vi "Recursive Model&Adaptive Control.vi"() -> ()   [LabVIEW 2015]
uses:
  <vilib>/addons/Control Design/_Model Construction/Model Typedefs.llb/CD State Space Model (MIMO).ctl
  <vilib>/addons/Control Design/_Model Construction/Model Typedefs.llb/CD General Elements.ctl
  <vilib>/addons/Control Design/_Stochastic Systems/Stochastic Systems.llb/Stochastic Systems SubVIs/cd_Second-Order Statistics Noise Model.ctl
  <vilib>/Platform/TimedLoop/XDataNode/timing_clust.ctl
  <vilib>/Platform/TimedLoop/XDataNode/nitl_modes.ctl
  <vilib>/Platform/TimedLoop/XDataNode/wakeup.ctl
  <vilib>/addons/Control Design/_Model Construction/Model Creation.llb/Model Creation SubVI/cd_Create State Space Model.vi
  <vilib>/FPGAPlugInAG/myRIO-1900/niLvFpga_Open_myRIO-1900.vi
  <vilib>/rvi/interface/common/dynamic/niFpgaDynamicAddResources.vi
  <vilib>/Utility/error.llb/Error Cluster From Error Code.vi
  <vilib>/rvi/errors/niLvFpgaAdjustHostInterfaceError.vi
  <vilib>/FPGAPlugInAG/Dynamic/niLvFpga_Close_Dynamic.vi
  <vilib>/addons/Control Design/_State Feedback Control/State Feedback Control.llb/State Feedback Control SubVis/cd_Kalman Gain (Stochastic).vi
  <vilib>/addons/Control Design/_State Feedback Control/State Feedback Control.llb/State Feedback Control SubVis/cd_Linear Quadratic Regulator.vi
  <vilib>/addons/Control Design/_State Feedback Control/State Feedback Control.llb/CD State Regulator.vi
  <vilib>/addons/Control Design/_Model Construction/Model Information.llb/Model Information SubVIs/cd_Get Matrices From SS Model.vi
  <vilib>/rvi/interface/nirviOpenFPGA/nirviOpenFPGA.xnode
  FPGA Bitfiles/ACC20115_FPGATarget_CurrentControlle_Dt5vFgOzYtY.lvbitx
  Current Controller.vi
  <vilib>/rvi/interface/nirviReadWriteControl/nirviReadWriteControl.xnode
  <vilib>/rvi/interface/nirviCloseFPGA/nirviCloseFPGA.xnode
  <vilib>/Platform/TimedLoop/XDataNode/XDataNode.xnode
  NiFpgaLv.dll
  <vilib>/rvi/interface/Simulation/niFpgaSimulationCallBeginRW.vi
  <vilib>/addons/Control Design/_Stochastic Systems/NI_CD_Stochastic Systems.lvlib
  <vilib>/Platform/TimedLoop/XDataNode/XDNodeRunTimeDep.lvlib
  <vilib>/addons/Control Design/_Model Construction/NI_LinSys_Model Creation.lvlib
  <vilib>/addons/Control Design/_State-Space Analysis/NI_CD_State-Space Analysis.lvlib
  <vilib>/addons/Control Design/_State Feedback Control/NI_CD_State Feedback Control.lvlib
  <vilib>/addons/Control Design/_Model Construction/NI_LinSys_Model Information.lvlib
  <vilib>/addons/Control Design/_Model Construction/NI_LinSys_Model Typedefs.lvlib
panel:
  out "error IO":errorcluster
  in  "Tab Control":enum32{"Outputs/Control", "Model Info"}(tab)
  out "DAC Inlet Valve 2":i32(graph)
  out "Fusion Data":dbl(graph)
  in  "Stop":bool
  out "FPGA Status?":bool
  in  "Current (mA)":i32
  out "Priori SS Detectable?":bool
  out "Priori SS Observable?":bool
  out "State-Space Model":T1 {"Transport Delay" format="%.2f"; "D" format="%#.2g"; "C" format="%#.2g"; "B" format="%#.2g"; "A" format="%#.2g"; "properties"."Sampling Time" format="%#.6p"; "properties"."Output Delays" format="%.4f"; "properties"."Input Delays" format="%.4f"}
  in  "A":dbl[][](array[numeric]) format="%#.5g"
  in  "B":dbl[][](array[numeric]) format="%#.5g"
  in  "C":dbl[][](array[numeric]) format="%#.5g"
  in  "D":dbl[][](array[numeric]) format="%#.5g"
  in  "G":dbl[][](array[numeric]) format="%#.2g"
  out "Riccati Solution (X)":dbl[][](array[numeric]) format="%.4f"
  in  "Noise Model":T3 {"N" format="%#.2g"; "R" format="%#.2g"; "E{v}" format="%#.2g"; "E{w}" format="%#.2g"; "Q" format="%#.2g"}
  out "error out":errorcluster
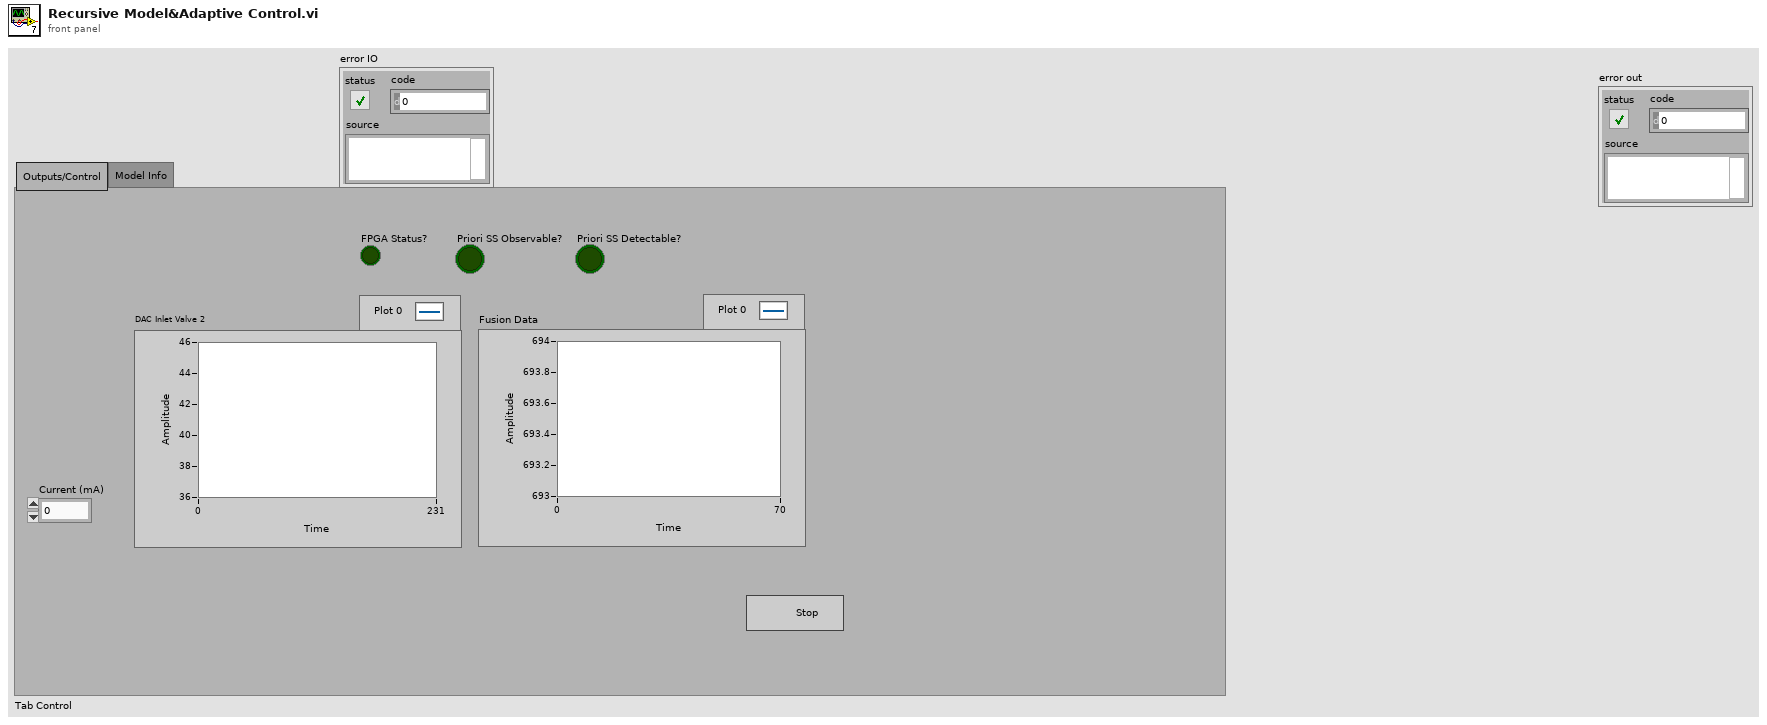
[diagram p1: front panel]
types:
  T1 = typedef "NI_LinSys_Model Typedefs.lvlib/CD State Space Model (MIMO).ctl" = cluster{"properties":T2, "A":dbl[][], "B":dbl[][], "C":dbl[][], "D":dbl[][], "StateNames":string[], "Transport Delay":dbl[][]}
  T2 = typedef "NI_LinSys_Model Typedefs.lvlib/CD General Elements.ctl" = cluster{"Model name":string, "Input names":string[], "Output names":string[], "Input Delays":dbl[], "Output Delays":dbl[], "Sampling Time":dbl, "Notes":string}
  T3 = typedef "NI_CD_Stochastic Systems.lvlib/cd_Second-Order Statistics Noise Model.ctl" = cluster{"Q":dbl[][], "E{w}":dbl[], "E{v}":dbl[], "R":dbl[][], "N":dbl[][]}
  T4 = typedef "XDNodeRunTimeDep.lvlib/timing_clust.ctl" = cluster{"Expected End [f-1]":u64, "Actual End [f-1]":u64, "Finished Late? [f-1]":bool, "Expected End [i-1]":u64, "Actual End [i-1]":u64, "Finished Late? [i-1]":bool, "Expected Start [i]":u64, "Actual Start [i]":u64, "Expected Start [f]":u64, "Actual Start [f]":u64, "Source Name":string, "Structure Name":string, "Period":i64, "Deadline":i64, "Offset":i64, "Start":i64, "Priority":i32, "Timeout":i32, "Mode":T5, "Wakeup Reason":T6, "Error":errorcluster, "Source Type":string, "Secondary Source Type":string, "Global End Time":u64, "Global Start Time":u64, "Frame Duration":u64, "Iteration Duration":u64, "Assigned CPU":i32, "I/O Scan Engine Mode":u32}
  T5 = typedef "XDNodeRunTimeDep.lvlib/nitl_modes.ctl" = enum32{"No Change", "Process missed periods, maintain original phase", "Discard missed periods, maintain original phase", "Process missed periods, ignore original phase", "Discard missed periods, ignore original phase"}
  T6 = typedef "XDNodeRunTimeDep.lvlib/wakeup.ctl" = enum32{"Normal", "Aborted", "Asynchronous wakeup", "Timing source error", "Timed loop error", "Timeout"}
  T7 = enum16{"System Included", "System Included with Noise", "Standalone"}
  T8 = enum16{"state weighting", "output weighting, Dim Q = Ny", "output weighting, Dim Q = Nx"}
  T9 = typedef "NI_CD_Stochastic Systems.lvlib/cd_Stochastic State-Space Model.ctl" = cluster{"Sampling Time (s)":dbl, "G":dbl[][], "B":dbl[][], "A":dbl[][], "C":dbl[][], "D":dbl[][], "H":dbl[][]}
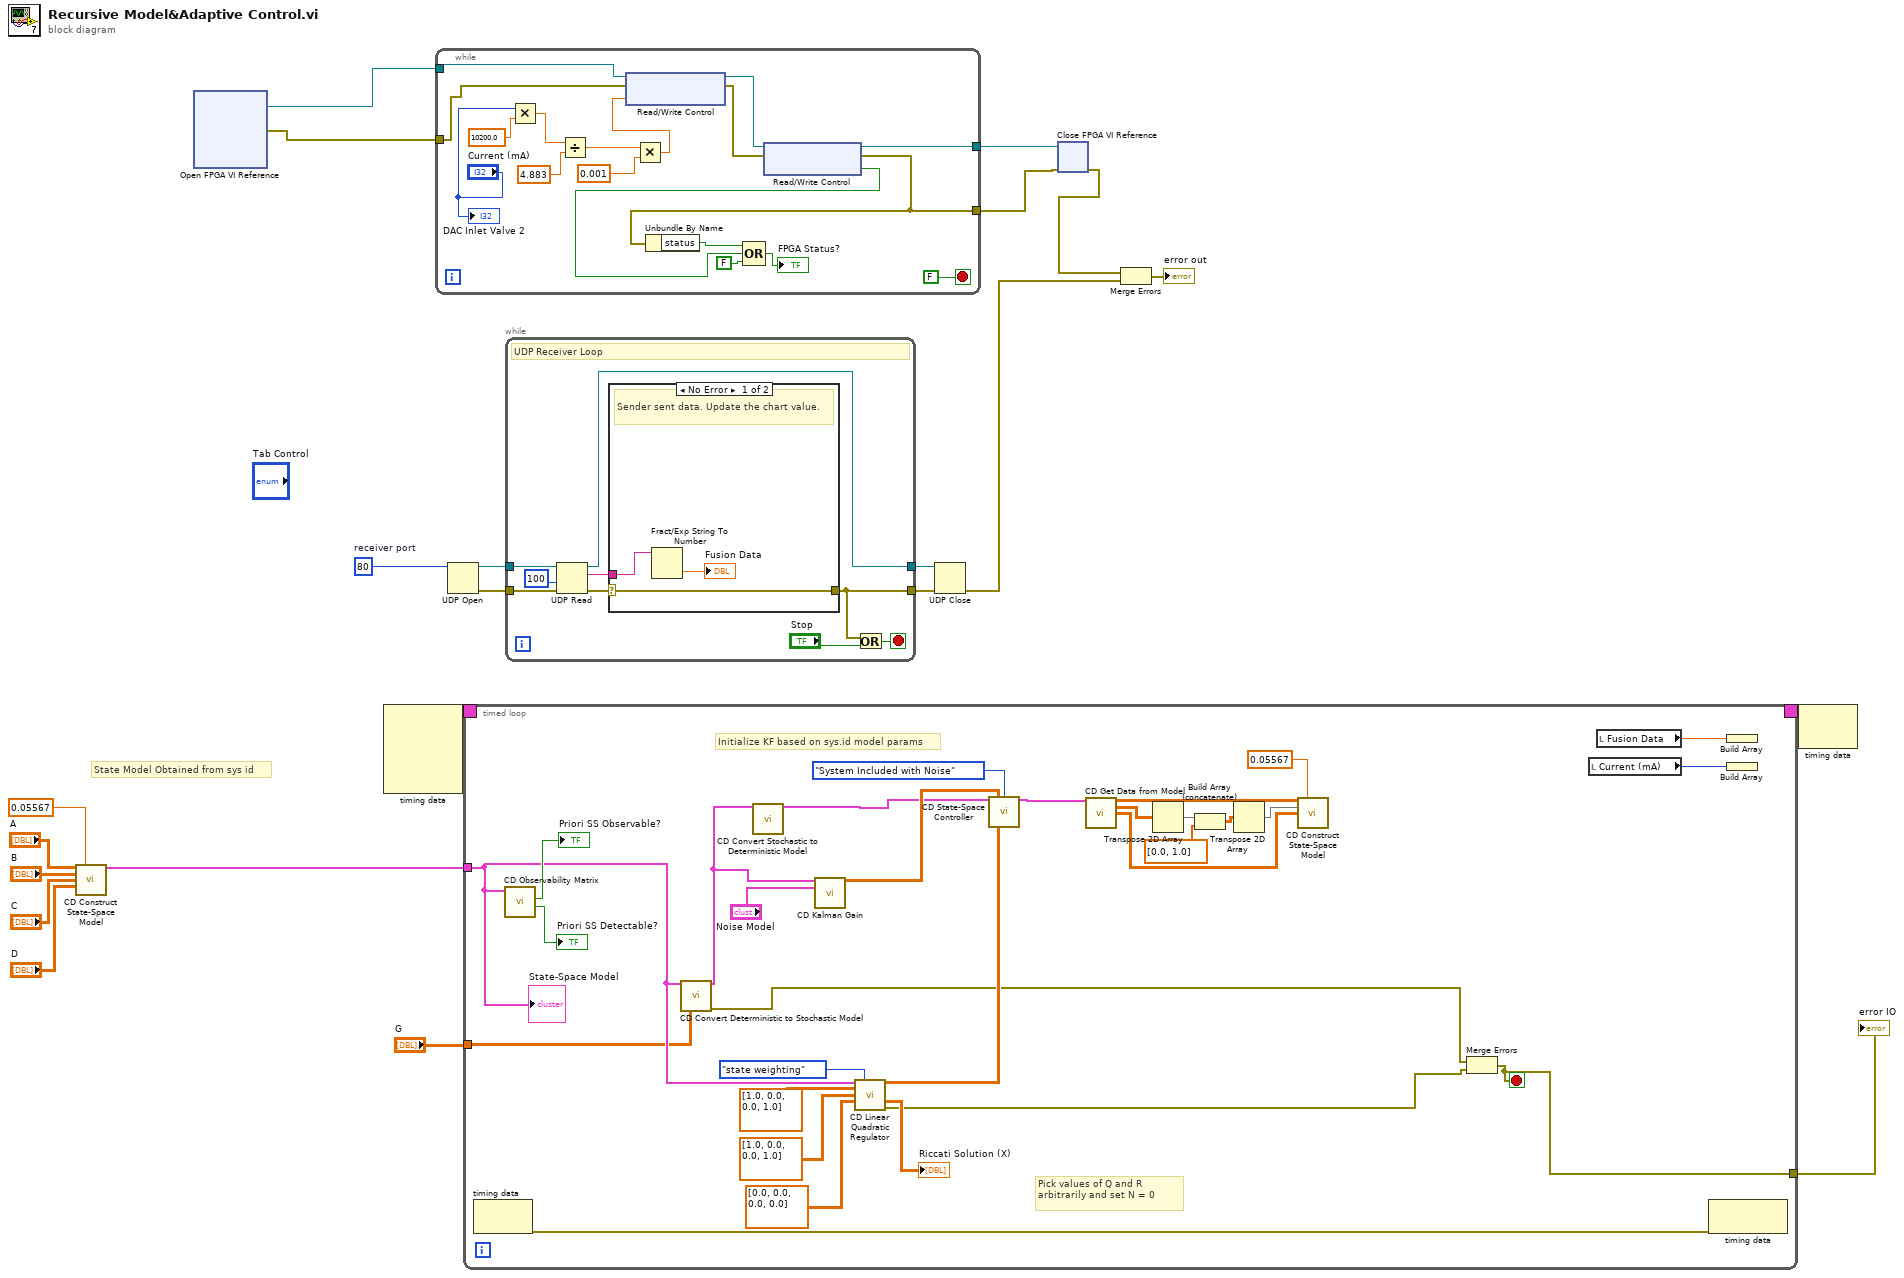
[diagram p0: block diagram]
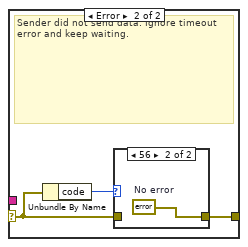
[diagram p2: hidden frame]
diagram:
  w18 = u16 80  # receiver port
  # "State Model Obtained from sys id"
  n1 = call-poly <vilib>:"CD Construct State-Space Model.vi"("A"="A", "Sampling Time (s)"=0.05567, "B"="B", "C"="C", "D"="D") -> ("State-Space Model"=w2:T1)  [unwired: 9 in, 1 out]
  n2 = xnode "Open FPGA VI Reference"() -> ("FPGA VI Reference Out"=w11:refnum<k20>, "error out"=w12:errorcluster)  [unwired: 2 in]
  n3 = node-c288() -> (w10:T4)  [unwired: 4 in]
  n4 = while {
    tunnel: w11 -> [w39]
    tunnel: w12 -> [w23]
    tunnel: [w33] -> w16
    tunnel: [w31] -> w17
    stop <- FALSE stop-if-true
    n5 = Multiply(x="Current (mA)", y=10200.0) -> (x*y=w26:dbl)
    n6 = Divide(x=w26, y=4.883) -> (x/y=w29:dbl)
    n7 = Multiply(x=w29, y=0.001) -> (x*y=w25:dbl)
    n8 = xnode "Read/Write Control"("FPGA VI Reference In"=w39, "error in"=w23, "DAC Inlet Valve"=w25) -> ("FPGA VI Reference Out"=w38:refnum<k20>, "error out"=w37:errorcluster)
    n9 = xnode "Read/Write Control"("FPGA VI Reference In"=w38, "error in"=w37) -> ("FPGA VI Reference Out"=w31:refnum<k20>, "error out"=w33:errorcluster, "Inlet Overflow?"=w32:bool)
    n10 = Unbundle By Name(w33) -> ("status"=w35:bool)
    n11 = Compound Arithmetic op=OR(w35, w32, FALSE ("value")) -> (→"FPGA Status?":bool)
    "DAC Inlet Valve 2" <- "Current (mA)"
  }
  n12 = UDP Open(11:w18) -> (port=w19:refnum<k16>, 0:w20:errorcluster)  [unwired: 4 in, 1 out]
  n13 = timed-loop {
    tunnel: [w67] -> w8
    timing: w10 -> [_]
    timing-out: [_] -> w9
    tunnel: w2 -> [w43]
    tunnel: "G" -> [w41]
    stop <- w67 stop-if-true
    # "Pick values of Q and R\narbitrarily and set N = 0"
    # "Initialize KF based on sys.id model params"
    n14 = node-c288() -> (w66:errorcluster)  [unwired: 1 in]
    n15 = call <vilib>:"CD Observability Matrix.vi"("State-Space Model"=w43) -> ("Is Detectable?"=→"Priori SS Detectable?":bool, "Is Observable?"=→"Priori SS Observable?":bool)  [unwired: 7 in, 2 out]
    n16 = call <vilib>:"CD Convert Deterministic to Stochastic Model.vi"("Deterministic State-Space Model"=w43, "G"=w41) -> ("Stochastic State-Space Model"=w47:T9, "error out"=w42:errorcluster)  [unwired: 12 in]
    n17 = call <vilib>:"CD Convert Stochastic to Deterministic Model.vi"("Stochastic State-Space Model"=w47) -> ("Deterministic State-Space Model"=w46:T1)  [unwired: 13 in, 1 out]
    n18 = call-poly <vilib>:"CD Kalman Gain.vi"("Stochastic State-Space Model"=w47, "Second-Order Statistics Noise Model"="Noise Model") -> ("Steady-State Kalman Gain (L)"=w59:dbl[][])  [unwired: 8 in, 5 out]
    n19 = call-poly <vilib>:"CD Linear Quadratic Regulator.vi"("State-Space Model"=w43, "Weighting Type"=T8."state weighting", "Q"=dbl[][] [[1.0, 0.0], [0.0, 1.0]], "R"=dbl[][] [[1.0, 0.0], [0.0, 1.0]], "N"=dbl[][] [[0.0, 0.0], [0.0, 0.0]]) -> ("Optimal Gain (K)"=w58:dbl[][], "Riccati Solution (X)"=→"Riccati Solution (X)":dbl[][], "error out"=w45:errorcluster)  [unwired: 7 in, 1 out]
    n20 = call-poly <vilib>:"CD State-Space Controller.vi"("State-Space Model"=w46, "Estimator Gain (L)"=w59, "Configuration"=T7."System Included with Noise", "Controller Gain (K)"=w58) -> ("Controller Model"=w50:T1)  [unwired: 10 in, 1 out]
    n21 = call-poly <vilib>:"CD Get Data from Model.vi"("State-Space Model"=w50) -> ("Matrix A"=w52:dbl[][], "Matrix B"=w57:dbl[][], "Matrix C"=w51:dbl[][])  [unwired: 10 in, 2 out]
    n22 = Transpose 2D Array(2D array=w57) -> (transposed array=w56:dbl[][])
    n23 = Build Array (concatenate)(w56, dbl[] [0.0, 1.0] ("sine wave")) -> (w54:dbl[][])
    n24 = Transpose 2D Array(2D array=w54) -> (transposed array=w53:dbl[][])
    n25 = call-poly <vilib>:"CD Construct State-Space Model.vi"("A"=w52, "Sampling Time (s)"=0.05567, "B"=w53, "C"=w51) -> ()  [unwired: 10 in, 2 out]
    n26 = Merge Errors(w42, w45) -> (w67:errorcluster)
    n27 = local read "Current (mA)"() -> (w69:i32)
    n28 = local read "Fusion Data"() -> (w70:dbl)
    n29 = node-c288(w66) -> ()  [unwired: 1 out]
    n30 = Build Array ("Build Array 6")(w70) -> ()  [unwired: 1 out]
    n31 = Build Array ("Build Array 5")(w69) -> ()  [unwired: 1 out]
    "State-Space Model" <- w43
  }
  "error IO" <- w8
  n32 = while {
    tunnel: w19 -> [w84]
    tunnel: [w76] -> w22
    tunnel: w20 -> [w81]
    tunnel: [w77] -> w21
    stop <- w82 stop-if-true
    # "UDP Receiver Loop"
    n33 = UDP Read(connection ID=w84, timeout ms (25000)=100, 8:w81) -> (data out=w79:string, error out=w78:errorcluster, 3:w76:refnum<k16>)  [unwired: 3 out]
    n34 = case shown="No Error" w78 {
      selector: w78 -> [w85 w89]
      tunnel: w79 -> [w87 _]
      tunnel: [w85 w88] -> w77
      frame No Error {
        # "Sender sent data. Update the chart value."
        n35 = Fract/Exp String To Number(string=w87) -> (number=→"Fusion Data":dbl)  [unwired: 3 in, 1 out]
      }
      frame Error {
        # "Sender did not send data. Ignore timeout error and keep waiting."
        n36 = Unbundle By Name(w89) -> ("code"=w90:i32)
        n37 = case shown="56" w90 {
          tunnel: w89 -> [w91 _]
          tunnel: [w91 w92] -> w88
          frame Default {
          }
          frame 56 {
            w92 = errorcluster {"status"=FALSE, "code"=0, "source"=""}  # No error
          }
        }
      }
    }
    n38 = Or(x=w77, y="Stop") -> (x .or. y?=w82:bool)
  }
  n39 = UDP Close(connection ID=w22, 8:w21) -> (error out=w14:errorcluster)  [unwired: 1 out]
  n40 = xnode "Close FPGA VI Reference"("FPGA VI Reference In"=w17, "error in"=w16) -> ("error out"=w15:errorcluster)
  n41 = Merge Errors(w15, w14) -> (→"error out":errorcluster)
  n42 = node-c288(w9) -> ()  [unwired: 1 out]
